vi "Associate Instruments to Paths.vi"(0 "Scalar SA Path Group in":refnum<class "SA 18GHz Path Group.lvclass">, 5 "TSM Context":T1, 11 "error in (no error)":errorcluster) -> (4 "Scalar SA Path Group out":refnum<class "SA 18GHz Path Group.lvclass">, 15 "error out":errorcluster)   [LabVIEW 2023, in "RFFixtureCharact.RFPM.lvlib" / "SA 18GHz Path Group.lvclass"]
uses:
  SA 18GHz Path Group.lvclass
  C:/srd-semi-rfcal-software/AuxTools/STSRFFixtureCharactUtility/Source/Code Modules/Common/Base Classes/Path Group/Path Group.lvclass
  <vilib>/NI_TestStand_SemiconductorModule/NI_TestStand_Semiconductor_Module.lvlibp/PinMap/General/SemiconductorModuleContext.ctl
  Paths/SA Path/SA 18GHz Path.lvclass
  C:/srd-semi-rfcal-software/AuxTools/STSRFFixtureCharactUtility/Source/Code Modules/Fixture/Public/Base Classes/Scalar/SA Abstract Path/SA Abstract Path.lvclass
  C:/srd-semi-rfcal-software/AuxTools/STSRFFixtureCharactUtility/Source/Code Modules/Common/Base Classes/Path/Path.lvclass
  C:/srd-semi-rfcal-software/AuxTools/STSRFFixtureCharactUtility/Source/Code Modules/Fixture/Public/Base Classes/Scalar/Scalar Path/Scalar Path.lvclass
  Charact Result Accessor/Scalar/Scalar Charact Result Accessor.lvclass
  C:/srd-semi-rfcal-software/AuxTools/STSRFFixtureCharactUtility/Source/Code Modules/Fixture/RFPM/Charact Result Accessor/Base/Charact Result Accessor.lvclass
  C:/srd-semi-rfcal-software/AuxTools/STSRFFixtureCharactUtility/Source/Code Modules/Common/Result Accessor/Result Accessor.lvclass
  Public/Base Classes/Scalar/SA Abstract Path/SA Abstract Path.lvclass/SA Abstract Path.ctl
  Public/Base Classes/Scalar/SA Abstract Path/Properties/Read Cal Tone Pin.vi
  Public/Base Classes/Scalar/SA Abstract Path/Properties/Write RFmx Session.vi
  <vilib>/NI_TestStand_SemiconductorModule/NI_TestStand_Semiconductor_Module.lvlibp/PinMap/RF/RFmx/PinToNIRFmxSession.vi
  <vilib>/NI_TestStand_SemiconductorModule/NI_TestStand_Semiconductor_Module.lvlibp/PinMap/RF/RFPM/PinToNIRFPMSessionsWithPaths.vi
  <vilib>/NI_TestStand_SemiconductorModule/NI_TestStand_Semiconductor_Module.lvlibp/PinMap/RF/RFSG/PinToNIRFSGSession.vi
  Common/Base Classes/Path/Path.lvclass
  Common/Result Accessor/Result Accessor.lvclass
  <vilib>/NI_TestStand_SemiconductorModule/NI_TestStand_Semiconductor_Module.lvlibp
  Common/Base Classes/Path Group/Path Group.lvclass
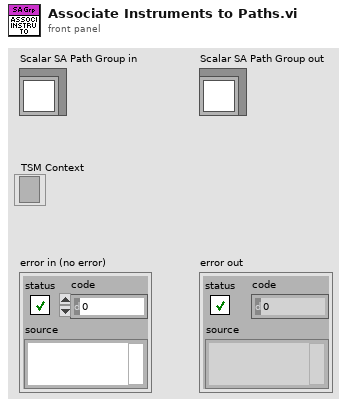
[diagram p1: front panel]
types:
  T1 = typedef "NI_TestStand_Semiconductor_Module.lvlibp/SemiconductorModuleContext.ctl" = refnum<k7>
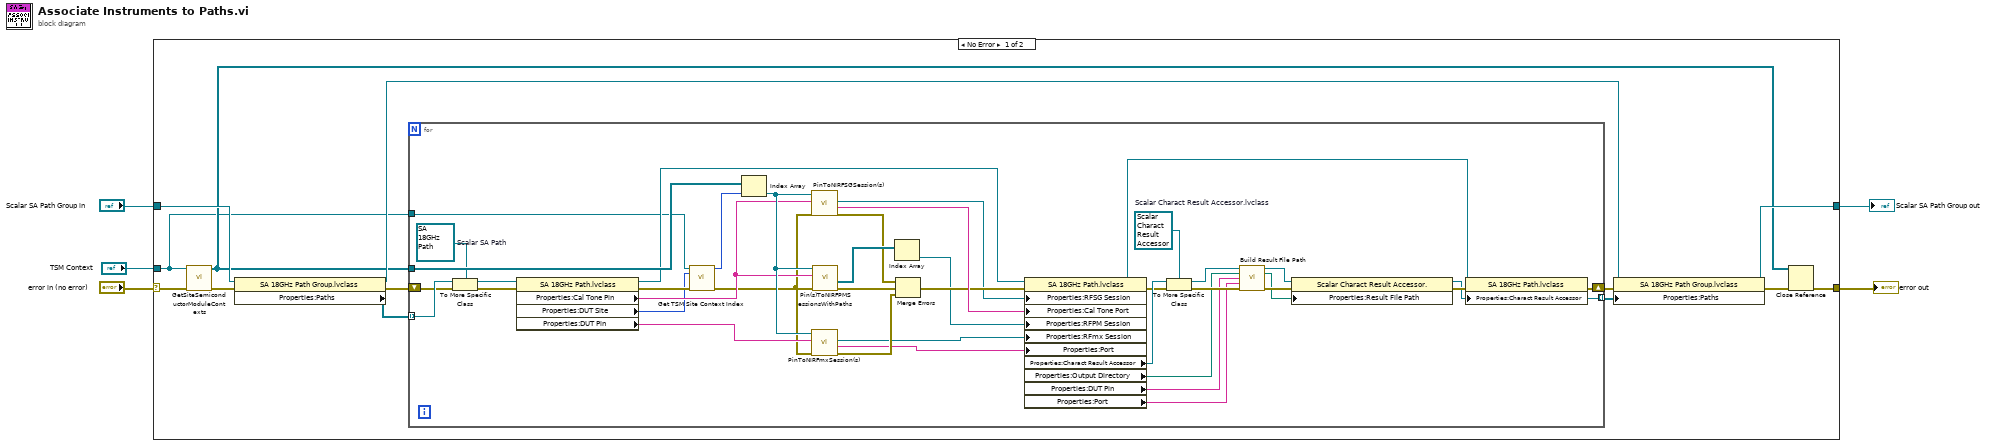
[diagram p0: block diagram]
diagram:
  n1 = case shown="No Error" "error in (no error)" {
    selector: "error in (no error)" -> [w7 w61]
    tunnel: "TSM Context" -> [w8 _]
    tunnel: "Scalar SA Path Group in" -> [w11 w60]
    tunnel: [w10 w61] -> w2
    tunnel: [w12 w60] -> w1
    frame No Error {
      n2 = call <vilib>:"GetSiteSemiconductorModuleContexts.vi"("error in (no error)"=w7, "Semiconductor Module Context"=w8) -> ("error out"=w16:errorcluster, "Site Semiconductor Module Contexts"=w9:T1[])  [unwired: 8 in]
      n3 = property class="SA 18GHz Path Group.lvclass"(reference=w11, error in=w16) -> (reference out=w14:refnum<class "SA 18GHz Path Group.lvclass">, error out=w6:errorcluster, "Properties:Paths"=w17:refnum<class "Path.lvclass">[])
      n4 = for {
        tunnel: w9 -> [w59]
        tunnel: w17 -> [w52] mode=indexing
        shift-right: [w31] -> w18
        shift-left: w6 -> [w47]
        tunnel: [w29] -> w13 mode=indexing
        tunnel: w8 -> [w37]
        w33 = refnum<class "Scalar Charact Result Accessor.lvclass"> refnum  # Scalar Charact Result Accessor.lvclass
        w48 = refnum<class "SA 18GHz Path.lvclass"> refnum  # Scalar SA Path
        n5 = To More Specific Class(target class=w48, reference=w52, error in=w47) -> (specific class reference=w49:refnum<class "SA 18GHz Path.lvclass">, error out=w46:errorcluster)
        n6 = property class="SA 18GHz Path.lvclass"(reference=w49, error in=w46) -> (reference out=w50:refnum<class "SA 18GHz Path.lvclass">, error out=w45:errorcluster, "Properties:Cal Tone Pin"=w39:string, "Properties:DUT Site"=w36:i32, "Properties:DUT Pin"=w43:string)
        n7 = call "Get TSM Site Context Index.vi"("Semiconductor Module Context"=w37, "Site Number"=w36, "error in (no error)"=w45) -> ("index of Site TSM Context"=w35:i32, "error out"=w38:errorcluster)  [unwired: 11 in]
        n8 = Index Array(array=w59, index=w35) -> (element=w44:T1)
        n9 = call-poly <vilib>:"PinToNIRFSGSession(s).vi"("error in (no error)"=w38, "Pin"=w39, "Semiconductor Module Context"=w44) -> ("error out"=w51:errorcluster, "Port"=w57:string, "Instrument Session"=w53:refnum<k15>)  [unwired: 4 in, 2 out]
        n10 = call-poly <vilib>:"PinToNIRFmxSession(s).vi"("error in (no error)"=w38, "Pin"=w43, "Semiconductor Module Context"=w44) -> ("error out"=w42:errorcluster, "Port"=w40:string, "Instrument Session"=w41:refnum<k21>)  [unwired: 4 in, 2 out]
        n11 = call-poly <vilib>:"Pin(s)ToNIRFPMSessionsWithPaths.vi"("error in (no error)"=w38, "Pin"=w39, "Semiconductor Module Context"=w44) -> ("error out"=w55:errorcluster, "Instrument Sessions"=w58:refnum<k15>[])  [unwired: 3 in, 4 out]
        n12 = Index Array(array=w58) -> (element=w54:refnum<k15>)  [unwired: 1 in]
        n13 = Merge Errors(w51, w55, w42) -> (w56:errorcluster)
        n14 = property class="SA 18GHz Path.lvclass"(reference=w50, error in=w56, "Properties:RFSG Session"=w53, "Properties:Cal Tone Port"=w57, "Properties:RFPM Session"=w54, "Properties:RFmx Session"=w41, "Properties:Port"=w40) -> (reference out=w27:refnum<class "SA 18GHz Path.lvclass">, error out=w28:errorcluster, "Properties:Charact Result Accessor"=w34:refnum<class "Result Accessor.lvclass">, "Properties:Output Directory"=w21:path, "Properties:DUT Pin"=w20:string, "Properties:Port"=w19:string)
        n15 = To More Specific Class(target class=w33, reference=w34, error in=w28) -> (specific class reference=w24:refnum<class "Scalar Charact Result Accessor.lvclass">, error out=w26:errorcluster)
        n16 = call-dynamic "Build Result File Path.vi"("Charact Result Accessor in"=w24, "Output Directory"=w21, "Port 1"=w20, "Port 2"=w19, "error in"=w26) -> ("Charact Result Accessor out"=w23:refnum<class "Scalar Charact Result Accessor.lvclass">, "Result File Path"=w22:path, "error out"=w25:errorcluster)  [unwired: 8 in]
        n17 = property class="Scalar Charact Result Accessor."(reference=w23, error in=w25, "Properties:Result File Path"=w22) -> (reference out=w30:refnum<class "Scalar Charact Result Accessor.lvclass">, error out=w32:errorcluster)
        n18 = property class="SA 18GHz Path.lvclass"(reference=w27, error in=w32, "Properties:Charact Result Accessor"=w30) -> (reference out=w29:refnum<class "SA 18GHz Path.lvclass">, error out=w31:errorcluster)
      }
      n19 = property class="SA 18GHz Path Group.lvclass"(reference=w14, error in=w18, "Properties:Paths"=w13) -> (reference out=w12:refnum<class "SA 18GHz Path Group.lvclass">, error out=w15:errorcluster)
      n20 = Close Reference(reference=w9, error in (no error)=w15) -> (error out=w10:errorcluster)
    }
    frame Error {
    }
  }
  "Scalar SA Path Group out" <- w1
  "error out" <- w2
